vi "lockintiempo.vi"() -> ()   [LabVIEW 2016]
panel:
  out "L/M":dbl(graph)
  in  "Lecturas":i32=1
  in  "Nombre del archivo":string
  in  "stop":bool
  in  "Delay(ms)":u32
  out "MULTIMETRO":dbl(graph)
  out "LOCK IN":dbl(graph)
  in  "Tipo":u16(ring)=1 items=["LockIn", "LockIn-DMM"]
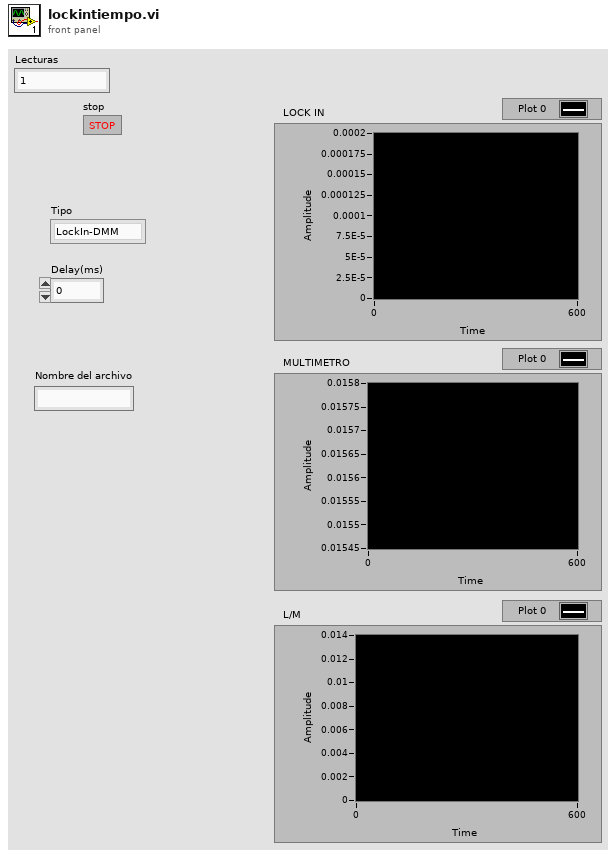
[diagram p1: front panel]
types:
  T1 = enum16{"Lockin", "Lockin-potenciometro", "Potenciometro"}
  T2 = enum16{"espejos", "polarizador", "voltaje", "potenciometro y lockin", "CCD"}
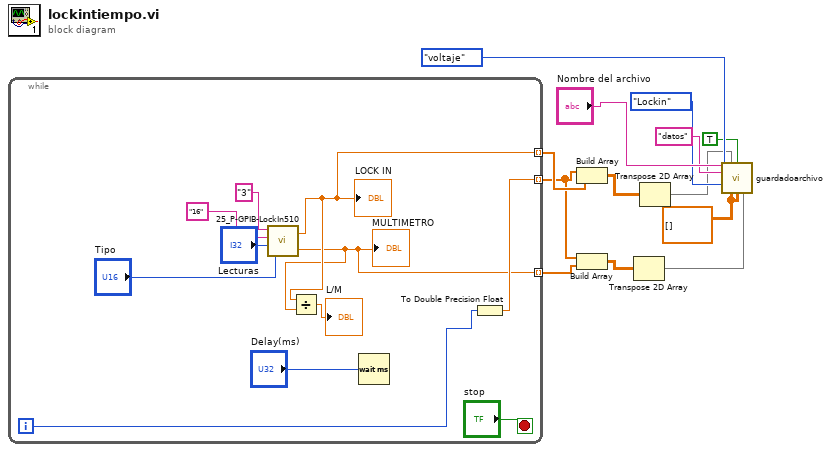
[diagram p0: block diagram]
diagram:
  w1 = dbl[][] [] ("polarizador")
  n1 = while {
    tunnel: [w15] -> w8 mode=indexing
    tunnel: [w18] -> w7 mode=indexing
    tunnel: [w14] -> w6 mode=indexing
    i -> [w19]
    stop <- "stop" stop-if-true
    n2 = call "25_P-GPIB-LockIn510.vi"("Tipo"="Tipo", "Lecturas"="Lecturas", "P-DMM"="16", "P-LockIn"="3") -> ("DMM"=w14:dbl, "LockIn"=w15:dbl)
    "LOCK IN" <- w15
    "MULTIMETRO" <- w14
    n3 = Divide(x=w15, y=w14) -> (x/y=→"L/M":dbl)
    n4 = Wait (ms)(milliseconds to wait="Delay(ms)") -> ()  [unwired: 1 out]
    n5 = To Double Precision Float(number=w19) -> (double precision float=w18:dbl)
  }
  n6 = Build Array(w7, w8) -> (w4:dbl[][])
  n7 = Build Array(w7, w6) -> (w5:dbl[][])
  n8 = Transpose 2D Array(2D array=w5) -> (transposed array=w2:dbl[][])
  n9 = Transpose 2D Array(2D array=w4) -> (transposed array=w3:dbl[][])
  n10 = call "guardadoarchivo.vi"("nombre"="Nombre del archivo", "lockin"=w3, "multimetro"=TRUE, "titulo grupo"="datos", "Tipo de Medición"=T1."Lockin", "element"=T2."voltaje", "polarizador"=w1, "corriente"=w1, "multim."=w2) -> ()  [unwired: 7 in]
